vi "sequencerCWTopLevel.vi"() -> ()   [LabVIEW 2014]
uses:
  Controls/measVoltState.ctl
  sequencerState.ctl
  Controls/SPstate.ctl
  Controls/heinzingerSelect.ctl
  Controls/triggerTypes.ctl
  Controls/selectTrigger.ctl
  Controls/triggerEdge.ctl
  OutBits/OutbitsStateControl.ctl
  <vilib>/rvi/Emulation/niFpgaGetClockAttributes.vi
  <vilib>/rvi/Emulation/niFpgaSctlEmulationGetInTimedLoop.vi
  <vilib>/rvi/Emulation/niFpgaEmulationReportErrorSimple.vi
  Trigger/triggerGlobalVars.vi
  <vilib>/rvi/Emulation/niFpgaProcessEmulError.vi
  ScanTrigger/scanTriggerGlobalVars.vi
  StepTrigger/stepTriggerGlobalVars.vi
  sequencerGlobVars.vi
  MeasVolt/measVoltGlobVars.vi
  QueueHandler/queueHandlerGlobals.vi
  SimpleCounter/SCGlobVars.vi
  HeinzingerControl/heinzingerControlGlobals.vi
  OutBits/OutbitsGlobalVars.vi
  <vilib>/rvi/Emulation/niFpgaCriticalErrorInLSC.vi
panel:
  in  "stepTrigDelay10ns":u32
  in  "softwareStepTrigger":bool
  in  "stepTriggerEdge":T1=enum."true-false"
  in  "stepTriggerTypes":T2
  in  "selectStepTrigger":T3
  in  "softwareScanTrigger":bool
  in  "scanTriggerEdge":T1=enum."true-false"
  in  "scanTrigDelay10ns":u32
  in  "selectScanTrigger":T3
  in  "scanTriggerTypes":T2
  out "nOfCmdsOutbit2":u32
  out "nOfCmdsOutbit1":u32
  out "nOfCmdsOutbit0":u32
  out "OutBitsState":T4
  in  "softwareTrigger":bool
  in  "pause":bool
  in  "stopVoltMeas":bool caption="measVoltStop"
  in  "measVoltCompleteDest":T5(ring)
  in  "dac0VRegister":u32=1572792 format="%024b"
  in  "triggerEdge":T1=enum."true-false"
  in  "trigDelay10ns":u32
  in  "selectTrigger":T3
  in  "triggerTypes":T2
  out "postAccOffsetVoltState":T6
  in  "postAccOffsetVoltControl":T6=enum."loading"
  out "SPerrorCount":u8
  out "SPstate":T7
  in  "dwellTime10ns":u32=2000000
  out "SPCtrQuWriteTimeout":bool
  in  "VoltOrScaler?":bool
  in  "dacStepSize18Bit":i32
  in  "dacStartRegister18Bit":i32
  in  "nOfSteps":i32
  in  "nOfScans":i32
  in  "invertScan":bool
  in  "waitForKepco(us)":u32
  in  "waitAfterReset(us)":u32 caption="waitForDmm(25nsTicks)"
  in  "measVoltPulseLength(25ns)":i32
  in  "measVoltTimeout(10ns)":i32 caption="measVoltTimeout(25ns)"
  in  "timedOutWhileHandshake":bool
  out "seqState":T8
  in  "cmdByHost":T8
  in  "abort":bool
  in  "halt":bool
  in  "hostConfirmsHzOffsetIsSet":bool
  out "measVoltState":T9
  out "DACQuWriteTimeout":bool
  # "Step Trigger"
  # "Step Trigger"
  # "Scan Trigger"
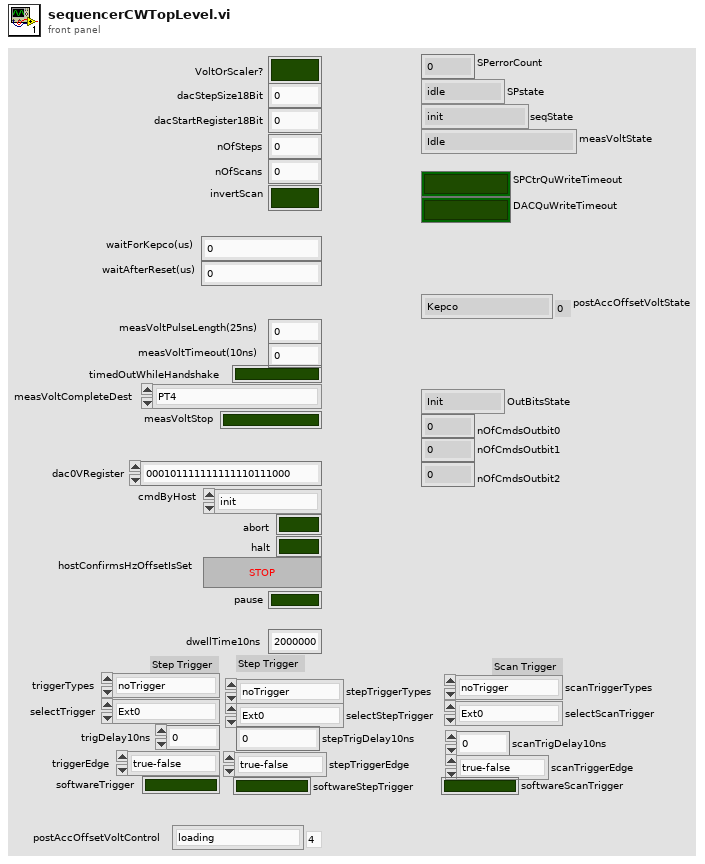
[diagram p1: front panel]
types:
  T1 = typedef "triggerEdge.ctl" = enum8{"either", "false-true", "true-false"}
  T2 = typedef "triggerTypes.ctl" = enum16{"noTrigger", "singleHitDelay", "singleHit", "software", "sweep"}
  T3 = typedef "selectTrigger.ctl" = enum8{"Ext0", "Ext1", "Ext2", "Ext3", "Ext4", "Ext5", "Ext6", "Ext7", "Int0", "Int1", "Int2", "Int3", "Int4", "Int5", "Int6", "Int7"}
  T4 = typedef "OutbitsStateControl.ctl" = enum16{"Init", "Idle", "loading", "listening", "clearing", "error"}
  T5 = enum16{"PT4", "C1D30", "C1D31", "PT4_C1D30", "PT4_C1D31", "PT4_C1D30_C1D31", "C1D30_C1D31"}
  T6 = typedef "heinzingerSelect.ctl" = enum8{"Kepco", "Heinzinger0", "Heinzinger1", "Heinzinger2", "loading"}
  T7 = typedef "SPstate.ctl" = enum16{"idle", "scanning", "done", "error"}
  T8 = typedef "sequencerState.ctl" = enum16{"init", "idle", "measureOffset", "measureTrack", "measComplete", "error"}
  T9 = typedef "measVoltState.ctl" = enum16{"Idle", "sendMeasRequest", "waitUntilDone", "done"}
  T10 = cluster{"SCLK":refnum<k21>, "CS":refnum<k21>, "MOSI":refnum<k21>, "MISO":refnum<k21>}
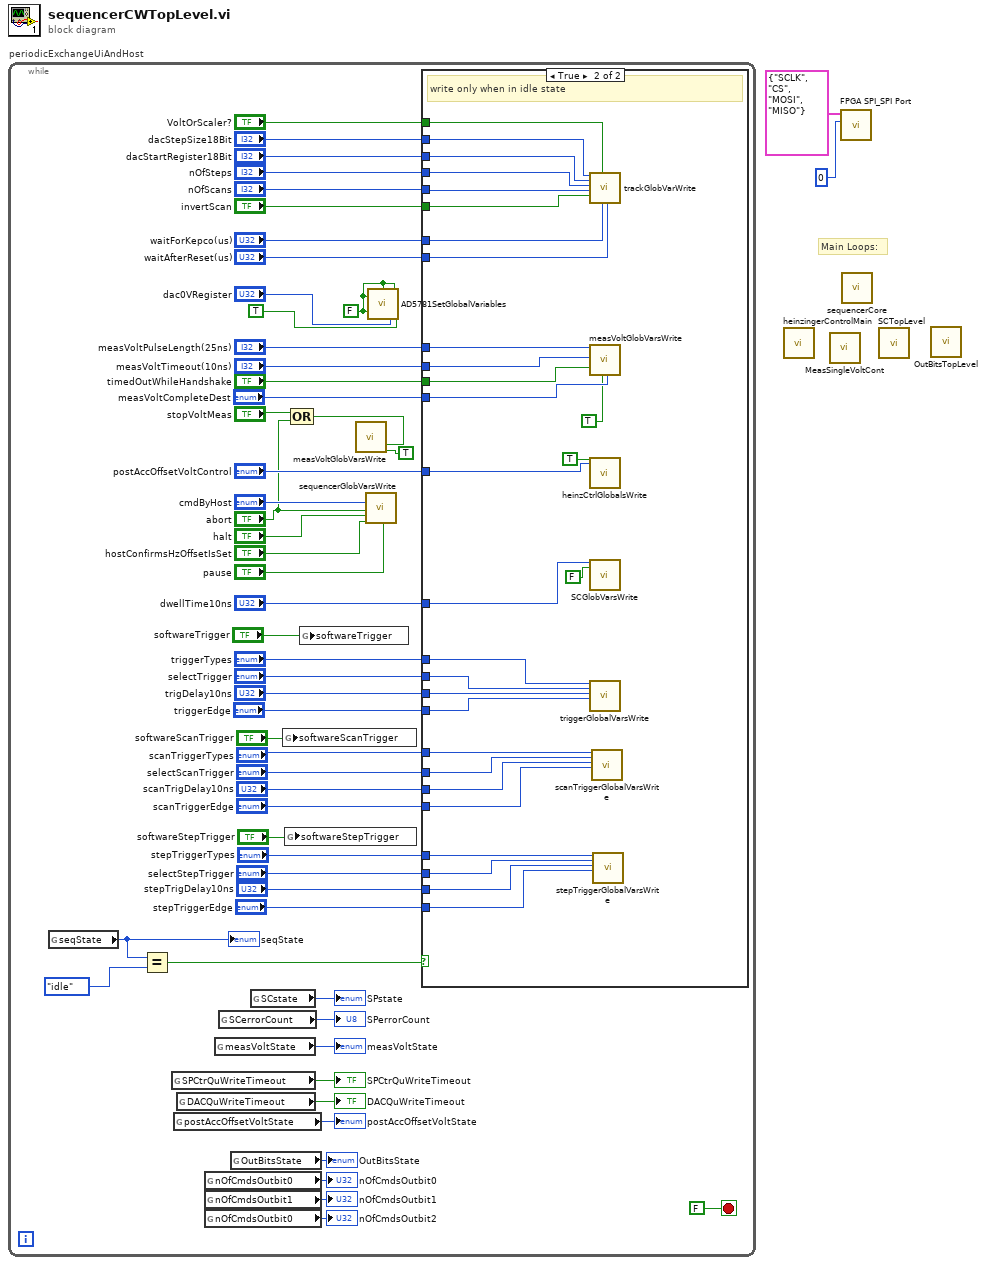
[diagram p0: block diagram]
diagram:
  # "Main Loops:"
  n1 = while "periodicExchangeUiAndHost" {
    stop <- FALSE stop-if-true
    w26 = FALSE ("write setDACRegister")
    n2 = global read "sequencerGlobVars.vi" "seqState"() -> (w38:T8)
    "seqState" <- w38
    n3 = Equal?(x=w38, y=sequencerState."idle") -> (x = y?=w55:bool)
    n4 = global read "queueHandlerGlobals.vi" "SPCtrQuWriteTimeout"() -> (→"SPCtrQuWriteTimeout":bool)
    n5 = global read "heinzingerControlGlobals.vi" "postAccOffsetVoltState"() -> (→"postAccOffsetVoltState":T6)
    n6 = global read "queueHandlerGlobals.vi" "DACQuWriteTimeout"() -> (→"DACQuWriteTimeout":bool)
    n7 = global read "OutbitsGlobalVars.vi" "nOfCmdsOutbit0"() -> (→"nOfCmdsOutbit0":u32)
    n8 = global read "OutbitsGlobalVars.vi" "nOfCmdsOutbit1"() -> (→"nOfCmdsOutbit1":u32)
    n9 = global read "OutbitsGlobalVars.vi" "nOfCmdsOutbit0"() -> (→"nOfCmdsOutbit2":u32)
    n10 = global read "measVoltGlobVars.vi" "measVoltState"() -> (→"measVoltState":T9)
    n11 = global read "SCGlobVars.vi" "SCerrorCount"() -> (→"SPerrorCount":u8)
    n12 = global read "OutbitsGlobalVars.vi" "OutBitsState"() -> (→"OutBitsState":T4)
    n13 = global read "SCGlobVars.vi" "SCstate"() -> (→"SPstate":T7)
    n14 = global write "scanTriggerGlobalVars.vi" "softwareScanTrigger"("softwareScanTrigger") -> ()
    n15 = global write "stepTriggerGlobalVars.vi" "softwareStepTrigger"("softwareStepTrigger") -> ()
    n16 = Compound Arithmetic op=OR("stopVoltMeas", "abort") -> (w20:bool)
    n17 = global write "triggerGlobalVars.vi" "softwareTrigger"("softwareTrigger") -> ()
    n18 = call "measVoltGlobVarsWrite.vi"("stopVoltMeas"=w20, "writeStopVoltMeas"=TRUE) -> ()  [unwired: 18 in]
    n19 = call "sequencerGlobVarsWrite.vi"("cmdByHost"="cmdByHost", "abort"="abort", "halt"="halt", "hostConfirmsHzOffsetIsSet"="hostConfirmsHzOffsetIsSet", "pause"="pause") -> ()  [unwired: 15 in]
    n20 = call "AD5781SetGlobalVariables.vi"("write actDACRegister"=w26, "write setDACRegister"=w26, "write DacStateCmdByHost"=w26, "dac0VRegister"="dac0VRegister", "writeSpiGlobals"=w26, "write dac0VRegister"=TRUE) -> ()  [unwired: 14 in]
    n21 = case shown="True" w55 {
      tunnel: "VoltOrScaler?" -> [_ w85]
      tunnel: "dacStepSize18Bit" -> [_ w84]
      tunnel: "dacStartRegister18Bit" -> [_ w83]
      tunnel: "nOfSteps" -> [_ w82]
      tunnel: "nOfScans" -> [_ w81]
      tunnel: "invertScan" -> [_ w80]
      tunnel: "waitForKepco(us)" -> [_ w79]
      tunnel: "waitAfterReset(us)" -> [_ w78]
      tunnel: "measVoltPulseLength(25ns)" -> [_ w77]
      tunnel: "measVoltTimeout(10ns)" -> [_ w76]
      tunnel: "timedOutWhileHandshake" -> [_ w75]
      tunnel: "dwellTime10ns" -> [_ w73]
      tunnel: "postAccOffsetVoltControl" -> [_ w71]
      tunnel: "triggerTypes" -> [_ w70]
      tunnel: "selectTrigger" -> [_ w69]
      tunnel: "trigDelay10ns" -> [_ w68]
      tunnel: "triggerEdge" -> [_ w67]
      tunnel: "measVoltCompleteDest" -> [_ w66]
      tunnel: "scanTriggerTypes" -> [_ w64]
      tunnel: "selectScanTrigger" -> [_ w63]
      tunnel: "scanTrigDelay10ns" -> [_ w62]
      tunnel: "scanTriggerEdge" -> [_ w61]
      tunnel: "stepTriggerTypes" -> [_ w60]
      tunnel: "selectStepTrigger" -> [_ w59]
      tunnel: "stepTrigDelay10ns" -> [_ w58]
      tunnel: "stepTriggerEdge" -> [_ w57]
      frame False {
      }
      frame True {
        # "write only when in idle state"
        n22 = call "trackGlobVarWrite.vi"("dacStepSize18Bit"=w84, "dacStartRegister18Bit"=w83, "nOfSteps"=w82, "nOfScans"=w81, "invertScan"=w80, "VoltOrScaler?"=w85, "waitForKepco(us)"=w79, "waitAfterReset(us)"=w78) -> ()  [unwired: 12 in]
        n23 = call "measVoltGlobVarsWrite.vi"("measVoltPulseLength(25ns)"=w77, "measVoltTimeout(10ns)"=w76, "timedOutWhileHandshake"=w75, "writeMeasVoltCompleteDest"=TRUE, "measVoltCompleteDest"=w66) -> ()  [unwired: 15 in]
        n24 = call "heinzCtrlGlobalsWrite.vi"("w_postAccOffsetVoltControl"=TRUE, "postAccOffsetVoltControl"=w71) -> ()  [unwired: 26 in]
        n25 = call "SCGlobVarsWrite.vi"("dwellTime10ns"=w73, "stop"=FALSE) -> ()  [unwired: 18 in]
        n26 = call "triggerGlobalVarsWrite.vi"("triggerTypes"=w70, "selectTrigger"=w69, "delay_10ns_ticks"=w68, "triggerEdge"=w67) -> ()  [unwired: 16 in]
        n27 = call "scanTriggerGlobalVarsWrite.vi"("scanTriggerTypes"=w64, "selectScanTrigger"=w63, "scan_trig_delay_10ns_ticks"=w62, "scanTriggerEdge"=w61) -> ()  [unwired: 16 in]
        n28 = call "stepTriggerGlobalVarsWrite.vi"("stepTriggerTypes"=w60, "selectStepTrigger"=w59, "step_trig_delay_10ns_ticks"=w58, "stepTriggerEdge"=w57) -> ()  [unwired: 16 in]
      }
    }
  }
  n29 = call "heinzingerControlMain.vi"() -> ()  [unwired: 3 in]
  n30 = call "MeasSingleVoltCont.vi"() -> ()  [unwired: 12 in]
  n31 = call "FPGA SPI_SPI Port.vi"("Port"=i8 0, "FPGA IO"=T10 {"SCLK"="SCLK", "CS"="CS", "MOSI"="MOSI", "MISO"="MISO"}) -> ()  [unwired: 10 in]
  n32 = call "sequencerCore.vi"() -> ()  [unwired: 12 in]
  n33 = call "SCTopLevel.vi"() -> ()  [unwired: 12 in]
  n34 = call "OutBitsTopLevel.vi"() -> ()  [unwired: 12 in]
